vi "Keep Array Size.vi"(10 "Size":i32, 11 "Array In":waveform(dbl)[](array[waveform])) -> (3 "Array Out":waveform(dbl)[](array[waveform]))   [LabVIEW 2021]
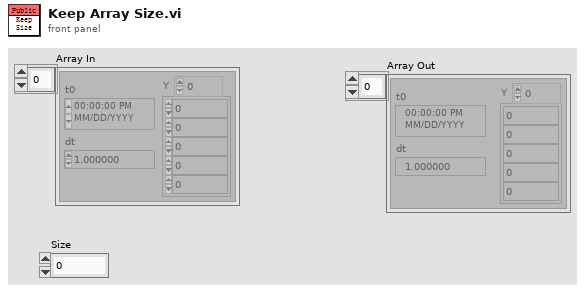
[diagram p1: front panel]
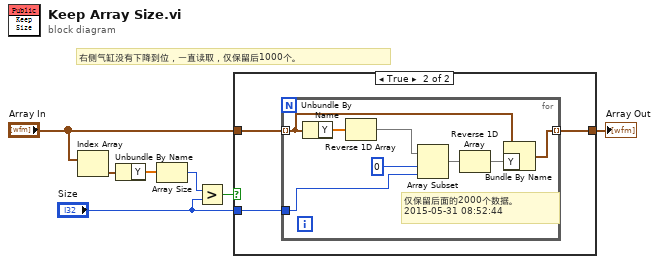
[diagram p0: block diagram]
diagram:
  # "右侧气缸没有下降到位，一直读取，仅保留后1000个。"
  n1 = Index Array(array="Array In") -> (element=w4:waveform(dbl))  [unwired: 1 in]
  n2 = Unbundle By Name(w4) -> ("Y"=w5:dbl[])
  n3 = Array Size(array=w5) -> (size(s)=w6:i32)
  n4 = Greater?(x=w6, y="Size") -> (0:w7:bool)
  n5 = case shown="True" w7 {
    tunnel: "Array In" -> [w8 w10]
    tunnel: [w8 w11] -> w1
    tunnel: "Size" -> [_ w9]
    frame False {
    }
    frame True {
      n6 = for {
        tunnel: w10 -> [w16] mode=indexing
        tunnel: [w14] -> w11 mode=indexing
        tunnel: w9 -> [w12]
        # "仅保留后面的2000个数据。\n2015-05-31 08:52:44"
        n7 = Unbundle By Name(w16) -> ("Y"=w19:dbl[])
        n8 = Reverse 1D Array(array=w19) -> (reversed array=w18:dbl[])
        n9 = Array Subset(array=w18, index=0, length=w12) -> (w15:dbl[])
        n10 = Reverse 1D Array(array=w15) -> (reversed array=w13:dbl[])
        n11 = Bundle By Name(cluster=w16, "Y"=w13) -> (w14:waveform(dbl))
      }
    }
  }
  "Array Out" <- w1
